vi "GetData.vi"(8 "error in (no error)":errorcluster, 10 "Data":T4, 11 "config in":T1) -> (0 "error out":errorcluster, 3 "config out":T1)   [LabVIEW 2017, in "TestPanel.lvlib"]
uses:
  <vilib>/addons/InsightCM/Devices/Shared/Common/TestPanel/TestPanel.lvlib
  <vilib>/addons/InsightCM/Devices/Shared/Common/TestPanel/controls/Configuration.ctl
  <vilib>/addons/InsightCM/Devices/Shared/Common/TestPanel/controls/State.ctl
  <vilib>/addons/InsightCM/MessageBus/Base/controls/IRoutingSource.ctl
  <vilib>/addons/InsightCM/Devices/Shared/Common/DataFlow/controls/Data.ctl
  <vilib>/addons/InsightCM/Utilities/DataAccessors/controls/wfmSGL_DVR.ctl
  <vilib>/addons/PointValueMap/controls/PointMap.ctl
  <vilib>/addons/InsightCM/Devices/Shared/Common/DataFlow/controls/Type.ctl
  <vilib>/addons/InsightCM/MessageBus/Base/controls/TestPanelTimeSeries.ctl
  <vilib>/addons/InsightCM/MessageBus/Base/controls/TestPanelValue.ctl
  <vilib>/addons/PointValueMap/subVIs/Point_Read_string.vi
  <vilib>/addons/PointValueMap/PointValueMap.lvlib
  <vilib>/addons/InsightCM/Devices/Shared/Common/DataFlow/DataFlow.lvlib
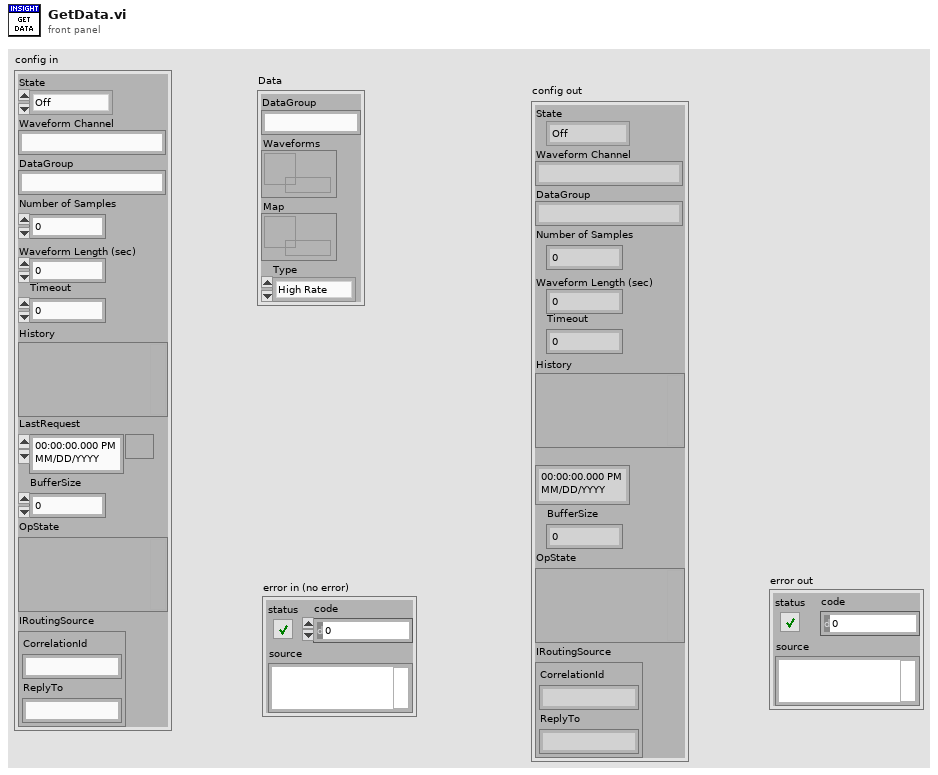
[diagram p1: front panel]
types:
  T1 = typedef "TestPanel.lvlib/Configuration.ctl" = cluster{"State":T2, "Waveform Channel":string, "DataGroup":string, "Number of Samples":i32, "Waveform Length (sec)":dbl, "Timeout":dbl, "History":variant, "LastRequest":timestamp, "BufferSize":i32, "OpState":variant, "IRoutingSource":T3}
  T2 = typedef "TestPanel.lvlib/State.ctl" = enum16{"Off", "On", "PendingValues", "PendingDataSet"}
  T3 = typedef "IRoutingSource.ctl" = cluster{"CorrelationId":string, "ReplyTo":string}
  T4 = typedef "DataFlow.lvlib/Data.ctl" = cluster{"DataGroup":string, "Waveforms":T5, "Map":T6, "Type":T7}
  T5 = typedef "wfmSGL_DVR.ctl" = refnum<data-value>
  T6 = typedef "PointValueMap.lvlib/PointMap.ctl" = refnum<data-value>
  T7 = typedef "DataFlow.lvlib/Type.ctl" = enum16{"High Rate", "Low Rate", "Burst Mode"}
  T8 = typedef "TestPanelTimeSeries.ctl" = cluster{"TrendPointId":string, "AssetName":string, "MetricName":string, "Unit":string, "Values":T9[]}
  T9 = typedef "TestPanelValue.ctl" = cluster{"Value":dbl, "Timestamp":i64, "Invalid":bool}
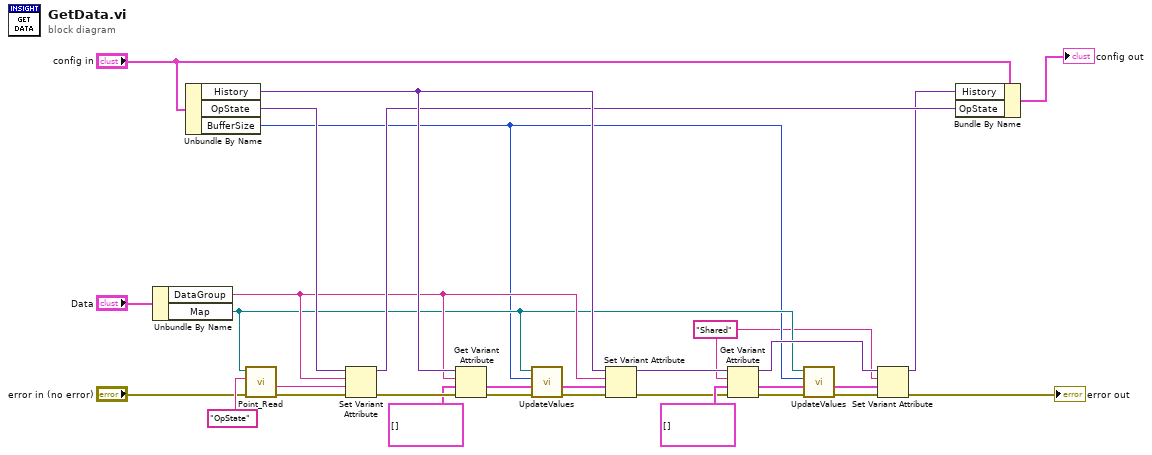
[diagram p0: block diagram]
diagram:
  w2 = "Shared" ("name")
  n1 = Unbundle By Name("Data") -> ("DataGroup"=w18:string, "Map"=w4:T6)
  n2 = Unbundle By Name("config in") -> ("History"=w28:variant, "OpState"=w27:variant, "BufferSize"=w3:i32)
  n3 = call-poly <vilib>:"Point_Read.vi"("Error In"="error in (no error)", "Tag"="OpState", "Map"=w4) -> ("Value"=w20:string)  [unwired: 3 in, 5 out]
  n4 = Set Variant Attribute(Variant=w27, name=w18, value=w20, error in="error in (no error)") -> (Variant out=w25:variant, error out=w21:errorcluster)  [unwired: 1 out]
  n5 = Get Variant Attribute(Variant=w28, name=w18, default value (empty Variant)=T8[] [], error in=w21) -> (value=w16:T8[], error out=w15:errorcluster)  [unwired: 2 out]
  n6 = call <vilib>:"UpdateValues.vi"("error in (no error)"=w15, "history values"=w16, "buffer size"=w3, "map"=w4) -> ("error out"=w22:errorcluster, "history values out"=w14:T8[])  [unwired: 6 in]
  n7 = Set Variant Attribute(Variant=w28, name=w18, value=w14, error in=w22) -> (Variant out=w6:variant, error out=w8:errorcluster)  [unwired: 1 out]
  n8 = Get Variant Attribute(Variant=w6, name=w2, default value (empty Variant)=T8[] [], error in=w8) -> (duplicate Variant=w5:variant, value=w11:T8[], error out=w12:errorcluster)  [unwired: 1 out]
  n9 = call <vilib>:"UpdateValues.vi"("error in (no error)"=w12, "history values"=w11, "buffer size"=w3, "map"=w4) -> ("error out"=w9:errorcluster, "history values out"=w13:T8[])  [unwired: 6 in]
  n10 = Set Variant Attribute(Variant=w5, name=w2, value=w13, error in=w9) -> (Variant out=w7:variant, error out=→"error out":errorcluster)  [unwired: 1 out]
  n11 = Bundle By Name(cluster="config in", "History"=w7, "OpState"=w25) -> (→"config out":T1)
